vi "ModbusTestRead.vi"() -> ()   [LabVIEW 2016]
uses:
  <vilib>/Instr/_visa.llb/VISA Configure Serial Port (Instr).vi
  <vilib>/NI Modbus.llb/MB Serial Master Query Read Holding Registers (poly).vi
panel:
  in  "VISA resource name":refnum<visa-resource-name>="COM4 (1)"
  out "Exception Code":u8 format="%.0x"
  out "error out":errorcluster
  out "Input Registers":u16[](array[numeric])
  in  "error in (no error)":errorcluster
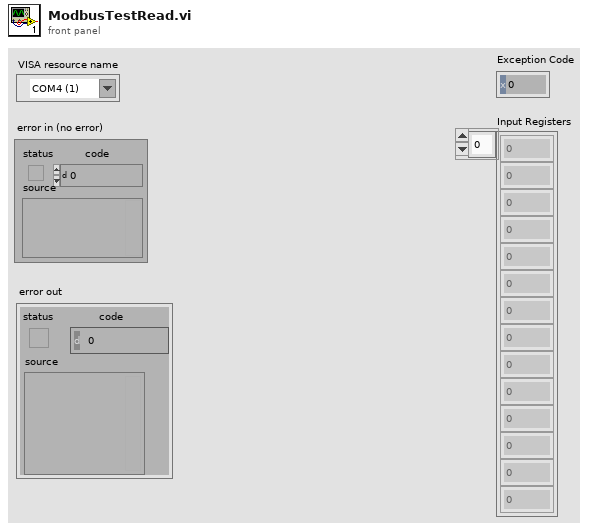
[diagram p1: front panel]
types:
  T1 = cluster{"Mode":enum16{"RTU", "ASCII"}, "Slave Address":u8}
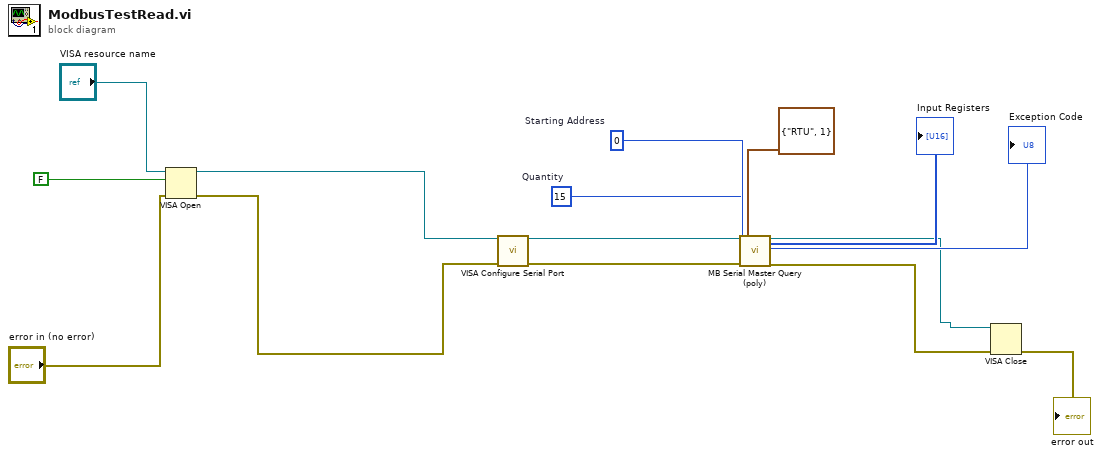
[diagram p0: block diagram]
diagram:
  w14 = u16 15  # Quantity
  w15 = u16 0  # Starting Address
  n1 = VISA Open(duplicate session (F)=FALSE, error in (no error)="error in (no error)", VISA resource name="VISA resource name") -> (VISA resource name=w8:refnum<visa-resource-name>, error out=w6:errorcluster)  [unwired: 2 in]
  n2 = call-poly "VISA Configure Serial Port"("VISA resource name"=w8, "error in (no error)"=w6) -> ("VISA resource name out"=w11:refnum<visa-resource-name>, "error out"=w4:errorcluster)  [unwired: 12 in]
  n3 = call-poly <vilib>:"MB Serial Master Query (poly).vi"("VISA resource name"=w11, "Starting Address"=w15, "Quantity"=w14, "error in"=w4, "Serial Parameters"=T1 {"Mode"=enum."RTU", "Slave Address"=1}) -> ("VISA resource name out"=w3:refnum<visa-resource-name>, "Holding Registers"=→"Input Registers":u16[], "Exception Code"=→"Exception Code":u8, "error out"=w2:errorcluster)  [unwired: 11 in]
  n4 = VISA Close(VISA resource name=w3, error in (no error)=w2) -> (error out=→"error out":errorcluster)
